vi "Macro Zip Load_Save.vi"(7 "Macro Zip Load_Save Command":T1, 8 "error in (no error)":errorcluster, 10 "Macro temp file path":path, 11 "source file path (*.sscr or *.zip)":path) -> (0 "error out":errorcluster, 1 "List of Settings Files in Temp":string[](array[string]), 2 "Macro File path OUT":path, 3 "Macro Text Out":string, 4 "Load Error?":bool)   [LabVIEW 2012]
doc: "SciScan 1.2 160622"
uses:
  Macro Zip Load_Save_Command.ctl
  <vilib>/zip/NI_Unzip.lvlib
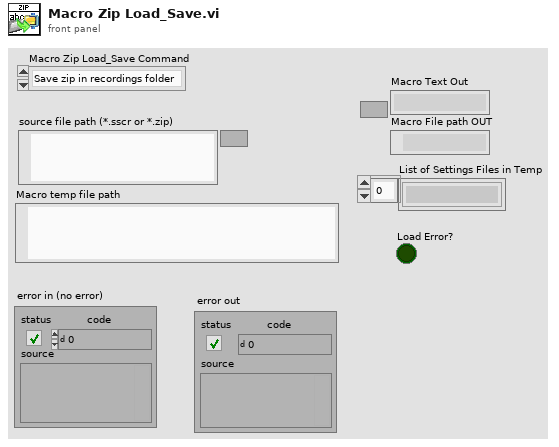
[diagram p1: front panel]
types:
  T1 = typedef "Macro Zip Load_Save_Command.ctl" = enum16{"Save zip in recordings folder", "Load macro from zip folder"}
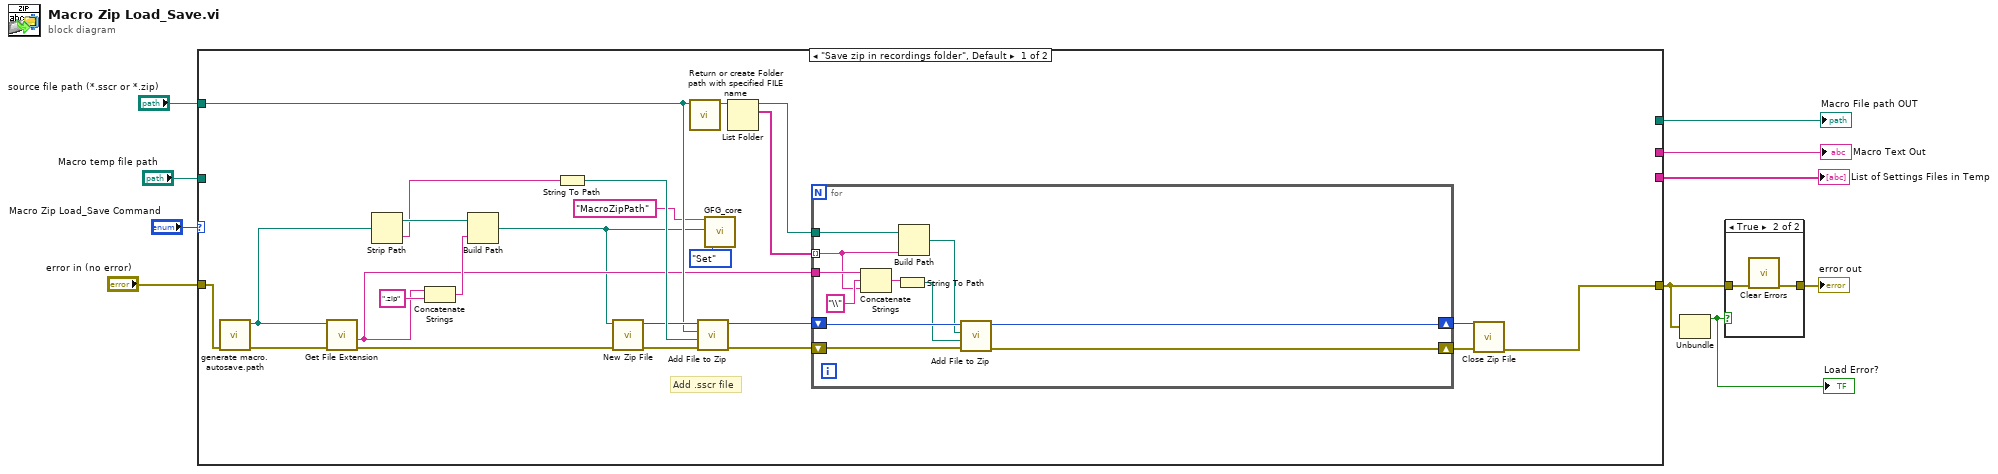
[diagram p0: block diagram]
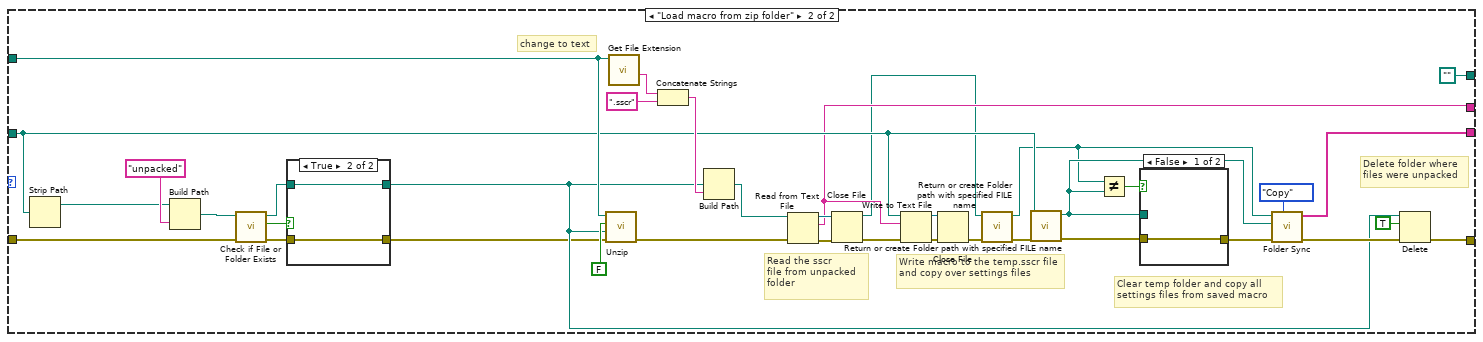
[diagram p3: hidden frame]
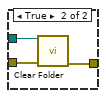
[diagram p4: hidden frame]
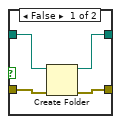
[diagram p5: hidden frame]
diagram:
  n1 = case shown="\"Save zip in recordings folder\", Default" "Macro Zip Load_Save Command" {
    tunnel: "source file path (*.sscr or *.zip)" -> [w24 w73]
    tunnel: "error in (no error)" -> [w16 w66]
    tunnel: [w14 w67] -> w5
    tunnel: "Macro temp file path" -> [_ w70]
    tunnel: [_ w49] -> w2
    tunnel: [_ path ""] -> w1
    tunnel: [_ w47] -> w3
    frame "Save zip in recordings folder", Default {
      # "Add .sscr file"
      n2 = call "generate macro.autosave.path.vi"("error in (no error)"=w16) -> ("error out"=w15:errorcluster, "macro.autosave.path"=w33:path)  [unwired: 9 in]
      n3 = call <vilib>:"Get File Extension.vi"("error in (no error)"=w15, "file"=w33) -> ("error out"=w34:errorcluster, "filename without extension"=w22:string)  [unwired: 6 in, 2 out]
      n4 = Strip Path(path=w33) -> (stripped path=w32:path, name=w29:string)
      n5 = Concatenate Strings(w22, ".zip" ("string")) -> (w30:string)
      n6 = Build Path(base path=w32, name or relative path=w30) -> (appended path=w11:path)
      n7 = String To Path(string=w29) -> (path=w28:path)
      n8 = call <vilib>:"New Zip File.vi"("error in (no error)"=w34, "target"=w11) -> ("error out"=w26:errorcluster, "zip file out"=w27:i64)  [unwired: 3 in, 1 out]
      n9 = call "Return or create Folder path with specified FILE name.vi"("File Path IN"=w24) -> ("Folder Path OUT"=w23:path)  [unwired: 9 in, 1 out]
      n10 = call <vilib>:"Add File to Zip.vi"("error in (no error)"=w26, "destination path in zip"=w28, "source file path"=w24, "zip file in"=w27) -> ("error out"=w25:errorcluster, "zip file out"=w20:i64)  [unwired: 6 in]
      n11 = call "GFG_core.vi"("Variable Name in"="MacroZipPath", "Variant in"=w11, "Action"=enum16{"Init", "Set", "Get", "Clear"}."Set") -> ()  [unwired: 10 in, 7 out]
      n12 = List Folder(path=w23) -> (path out=w19:path, filenames=w21:string[])  [unwired: 3 in, 2 out]
      n13 = for {
        tunnel: w22 -> [w44]
        tunnel: w21 -> [w37] mode=indexing
        shift-right: [w40] -> w17
        shift-left: w20 -> [w41]
        tunnel: w19 -> [w38]
        shift-right: [w35] -> w18
        shift-left: w25 -> [w45]
        n14 = Concatenate Strings(w44, "\\" ("string"), w37) -> (w42:string)
        n15 = String To Path(string=w42) -> (path=w39:path)
        n16 = Build Path(base path=w38, name or relative path=w37) -> (appended path=w36:path)
        n17 = call <vilib>:"Add File to Zip.vi"("error in (no error)"=w45, "destination path in zip"=w39, "source file path"=w36, "zip file in"=w41) -> ("error out"=w35:errorcluster, "zip file out"=w40:i64)  [unwired: 6 in]
      }
      n18 = call <vilib>:"Close Zip File.vi"("error in (no error)"=w18, "zip file in"=w17) -> ("error out"=w14:errorcluster)  [unwired: 5 in]
    }
    frame "Load macro from zip folder" {
      # "Write macro to the temp.sscr file and copy over settings files"
      # "Read the sscr\nfile from unpacked\nfolder"
      # "Clear temp folder and copy all \nsettings files from saved macro"
      # "Delete folder where\nfiles were unpacked"
      # "change to text"
      n19 = Strip Path(path=w70) -> (stripped path=w78:path)  [unwired: 1 out]
      n20 = Build Path(base path=w78, name or relative path="unpacked") -> (appended path=w76:path)
      n21 = call <vilib>:"Check if File or Folder Exists.vi"("error in (no error)"=w66, "path"=w76) -> ("error out"=w74:errorcluster, "file or folder exists?"=w77:bool, "dup path"=w75:path)  [unwired: 7 in]
      n22 = case shown="True" w77 {
        tunnel: w75 -> [w90 w92]
        tunnel: [w89 w92] -> w68
        tunnel: w74 -> [w88 w91]
        tunnel: [w87 w91] -> w65
        frame False {
          n23 = Create Folder(path (use dialog)=w90, error in=w88) -> (created path=w89:path, error out=w87:errorcluster)  [unwired: 1 in, 1 out]
        }
        frame True {
        }
      }
      n24 = call <vilib>:"Unzip.vi"("error in (no error)"=w65, "Target directory (same as Zip file if empty)"=w68, "Preview only?"=FALSE, "Zip file"=w73) -> ("error out"=w64:errorcluster)  [unwired: 5 in, 2 out]
      n25 = call <vilib>:"Get File Extension.vi"("file"=w73) -> ("filename without extension"=w81:string)  [unwired: 7 in, 3 out]
      n26 = Concatenate Strings(w81, ".sscr" ("string")) -> (w72:string)
      n27 = Build Path(base path=w68, name or relative path=w72) -> (appended path=w71:path)
      n28 = Read from Text File(file (use dialog)=w71, error in=w64) -> (refnum out=w61:refnum<file>, text=w49:string, error out=w62:errorcluster)  [unwired: 2 in, 1 out]
      n29 = Close File(refnum=w61, error in=w62) -> (path=w48:path, error out=w60:errorcluster)
      n30 = Write to Text File(file (use dialog)=w70, text=w49, error in=w60) -> (refnum out=w58:refnum<file>, error out=w59:errorcluster)  [unwired: 1 in, 1 out]
      n31 = Close File(refnum=w58, error in=w59) -> (error out=w55:errorcluster)  [unwired: 1 out]
      n32 = call "Return or create Folder path with specified FILE name.vi"("error in (no error)"=w55, "File Path IN"=w48) -> ("error out"=w54:errorcluster, "Folder Path OUT"=w51:path)  [unwired: 8 in]
      n33 = call "Return or create Folder path with specified FILE name.vi"("error in (no error)"=w54, "File Path IN"=w70) -> ("error out"=w53:errorcluster, "Folder Path OUT"=w52:path)  [unwired: 8 in]
      n34 = Not Equal?(x=w51, y=w52) -> (x != y?=w50:bool)
      n35 = case shown="False" w50 {
        tunnel: [w83 w86] -> w56
        tunnel: w53 -> [w83 w85]
        tunnel: w52 -> [_ w84]
        frame False {
        }
        frame True {
          n36 = call "Clear Folder.vi"("error in (no error)"=w85, "Path"=w84) -> ("error out"=w86:errorcluster)  [unwired: 9 in]
        }
      }
      n37 = call "Folder Sync.vi"("Copy(default)/Move"=enum16{"Copy", "Move"}."Copy", "error in (no error)"=w56, "Destination Folder (To be modified)"=w52, "Source Folder"=w51) -> ("error out"=w69:errorcluster, "List of Files Copied/Moved"=w47:string[])  [unwired: 6 in]
      n38 = Delete(path (use dialog)=w68, entire hierarchy (F)=TRUE, error in=w69) -> (error out=w67:errorcluster)  [unwired: 2 in, 2 out]
    }
  }
  "List of Settings Files in Temp" <- w3
  "Macro Text Out" <- w2
  "Macro File path OUT" <- w1
  n39 = Unbundle(w5) -> ("status"=w6:bool)  [unwired: 2 out]
  "Load Error?" <- w6
  n40 = case shown="True" w6 {
    tunnel: w5 -> [w93 w95]
    tunnel: [w93 w94] -> w4
    frame False {
    }
    frame True {
      n41 = call <vilib>:"Clear Errors.vi"("error in (no error)"=w95) -> ("error out"=w94:errorcluster)  [unwired: 6 in]
    }
  }
  "error out" <- w4
